vi "AsyncActor.vi"(7 "Actor":refnum<class "Actor.lvclass">) -> (0 "Error":errorcluster)   [LabVIEW 2020, in "jettl.lvlib"]
uses:
  jettl.lvlib
  Actor/Actor.lvclass
  Actor.vi
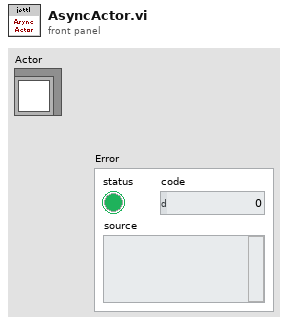
[diagram p1: front panel]
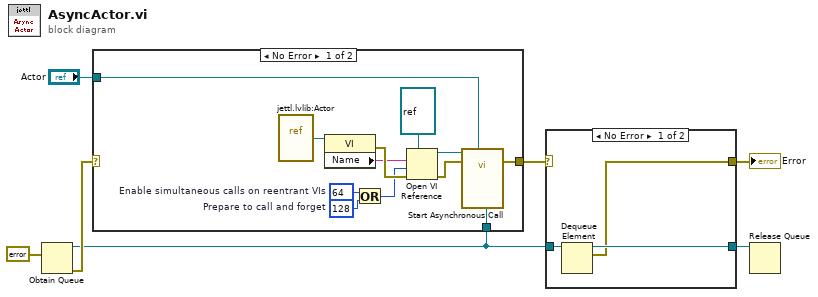
[diagram p0: block diagram]
diagram:
  n1 = Obtain Queue(element data type=errorcluster {"status"=FALSE, "code"=0, "source"=""} ("Error")) -> (queue out=w3:refnum<queue>, error out=w7:errorcluster)  [unwired: 4 in, 1 out]
  n2 = case shown="No Error" w7 {
    selector: w7 -> [_ w20]
    tunnel: [w10 w20] -> w5
    tunnel: "Actor" -> [w8 _]
    tunnel: w3 -> [w9 _]
    frame No Error {
      w14 = 64  # Enable simultaneous calls on reentrant VIs
      w15 = 128  # Prepare to call and forget
      n3 = vi-ref "jettl.lvlib:Actor.vi"() -> (w17:refnum<vi>)
      n4 = property class="VI"(reference=w17) -> (error out=w19:errorcluster, "Name"=w18:string)  [unwired: 1 in, 1 out]
      n5 = Or(x=w14, y=w15) -> (x .or. y?=w13:i32)
      n6 = Open VI Reference(type specifier VI Refnum (for type only)=refnum<vi> refnum, vi path=w18, options=w13, error in (no error)=w19) -> (vi reference=w12:refnum<vi>, error out=w11:errorcluster)  [unwired: 2 in]
      n7 = call-by-ref "Start Asynchronous Call"(reference=w12, error in=w11, "ErrorQueue"=w9, "Actor in"=w8) -> (error out=w10:errorcluster)  [unwired: 8 in, 3 out]
    }
    frame Error {
    }
  }
  n8 = case shown="No Error" w5 {
    selector: w5 -> [_ w25]
    tunnel: w3 -> [w23 w24]
    tunnel: [w21 w25] -> w6
    tunnel: [w22 w24] -> w1
    frame No Error {
      n9 = Dequeue Element(queue=w23) -> (queue out=w22:refnum<queue>, element=w21:errorcluster)  [unwired: 2 in, 2 out]
    }
    frame Error {
    }
  }
  "Error" <- w6
  n10 = Release Queue(queue=w1) -> ()  [unwired: 2 in, 3 out]
